vi "event.create_programmatic.request.vi"(4 "Additional Information":T1, 5 "Duration (0s)":dbl, 6 "Properties and Labels":T2, 7 "Time Stamp (now: system time)":timestamp format="%<%x %.3X>T", 8 "error in":errorcluster, 9 "Name":string, 10 "Asset RIDs":string[](array[string])) -> (0 "error out":errorcluster, 3 "request":string)   [LabVIEW 2020, in "Nominal Client.lvclass"]
uses:
  Nominal Client.lvclass
  762c8870-e4d3-421c-a376-3e8bab40d908.vi
  a7848146-fc71-4dc3-8a34-870616c71ff8.vi
  7e86f393-abb9-4d64-98a3-bbc5c32f8c9f.vi
  adfb2873-4f8f-45ec-91b4-e6f8d4ca100d.vi
  f3b2abde-4779-4471-9147-3371a6e54b37.vi
  a6a03f40-2490-4db4-85a0-99c3ddd96217.vi
  <vilib>/LabVIEW Open Source Project/Epoch Date & Time/epoch.UNIX/Epoch.UNIX.lvclass
  C:/Program Files/National Instruments/LabVIEW 2020/vi.lib/LabVIEW Open Source Project/Epoch Date & Time/epoch/Epoch.lvclass
  <vilib>/LabVIEW Open Source Project/Epoch Date & Time/Get Epoch Time.vi
  <vilib>/JDP Science/JSONtext/Variant to JSON Text.vi
  <vilib>/JDP Science/JSONtext/support/Format JSON Object.vi
  <vilib>/JDP Science/JSONtext/LVClass Serializer/JSONtext LVClass Serializer.lvclass
  nominal types/labels/labels.lvclass
  Nominal Client.lvclass/Nominal Client.ctl
  nominal types/properties/properties.lvclass
  <vilib>/JDP Science/JSONtext/JSONtext.lvlib
  133ea0b1-5c8c-48d2-80aa-f88861def257.vi
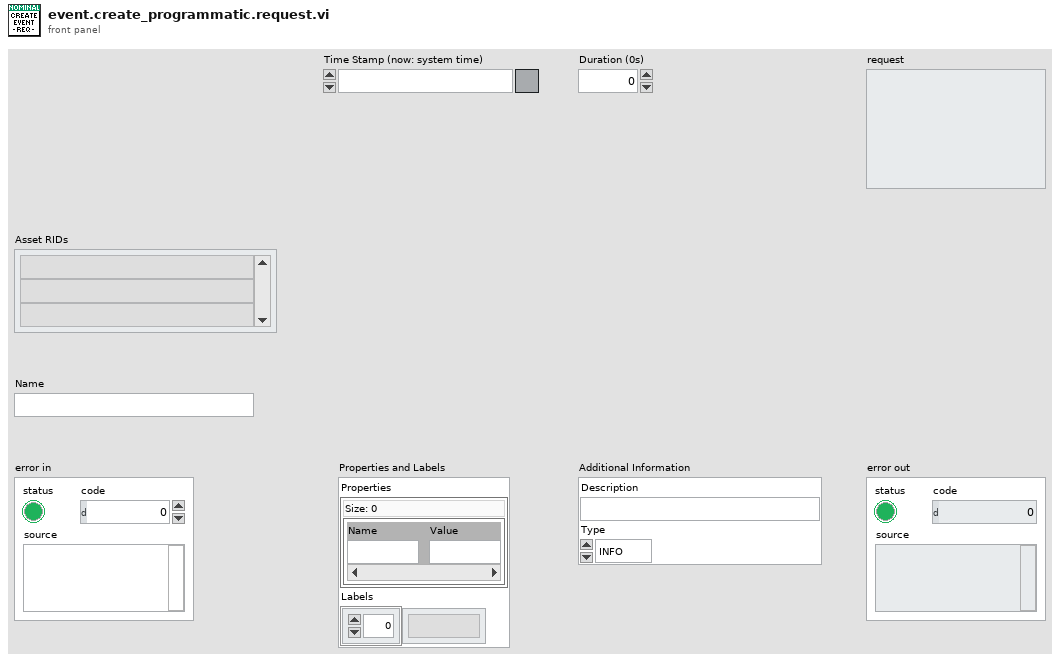
[diagram p1: front panel]
types:
  T1 = cluster{"Description":string, "Type":enum16{"INFO", "FLAG", "ERROR", "SUCCESS"}}
  T2 = cluster{"Properties":map{string, string}, "Labels":string[]}
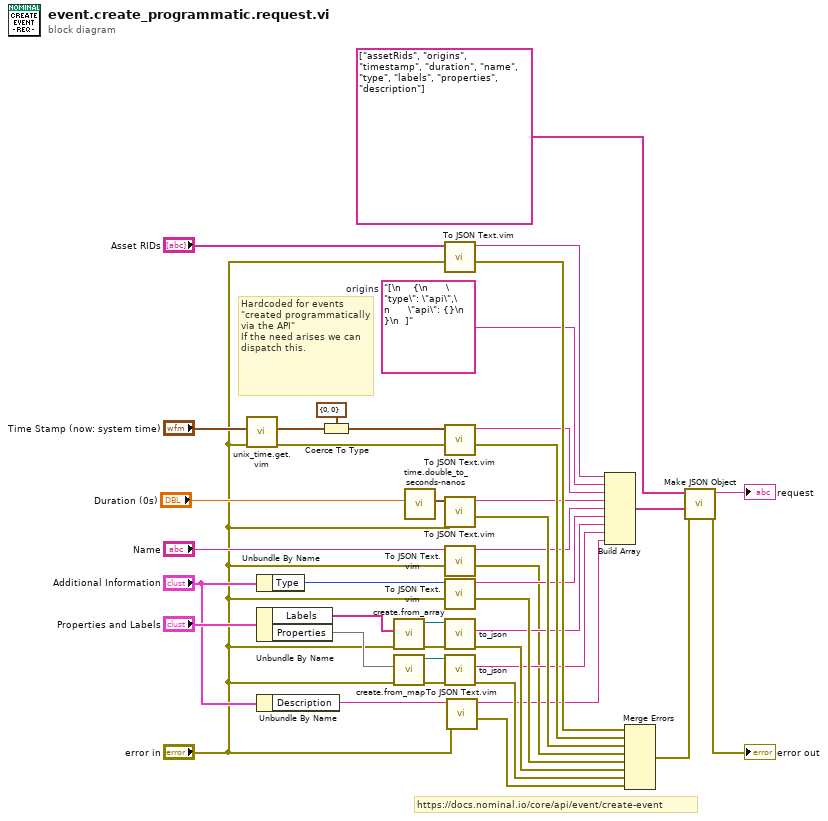
[diagram p0: block diagram]
diagram:
  w22 = "[\n    {\n      \"type\": \"api\",\n      \"api\": {}\n    }\n  ]"  # origins
  # "Hardcoded for events \"created programmatically via the API\"\nIf the need arises we can dispatch this."
  # "https://docs.nominal.io/core/api/event/create-event"
  n1 = call "unix_time.get.vim"("Time Stamp (empty: now) [single or array]"="Time Stamp (now: system time)") -> ("UNIX Timestamp"=w40:cluster{"Seconds":i64, "Nanoseconds":i64})  [unwired: 10 in]
  n2 = Unbundle By Name("Additional Information") -> ("Type"=w6:enum16{"INFO", "FLAG", "ERROR", "SUCCESS"})
  n3 = Unbundle By Name("Properties and Labels") -> ("Labels"=w34:string[], "Properties"=w36:map{string, string})
  n4 = Unbundle By Name("Additional Information") -> ("Description"=w4:string)
  n5 = Coerce To Type(0:w40, 1:cluster{"seconds":i32, "nanos":i32} {"seconds"=0, "nanos"=0} ("UNIX Timestamp")) -> (2:w29:cluster{"seconds":i32, "nanos":i32})
  n6 = call "create.from_array.vi"("error in"="error in", "labels"=w34) -> ("error out"=w32:errorcluster, "labels out"=w33:refnum<class "labels.lvclass">)  [unwired: 8 in]
  n7 = call "create.from_map.vi"("error in"="error in", "properties"=w36) -> ("error out"=w31:errorcluster, "properties out"=w35:refnum<class "properties.lvclass">)  [unwired: 8 in]
  n8 = call "time.double_to_seconds-nanos.vi"("Time (s)"="Duration (0s)") -> ("Seconds Nanos"=w15:cluster{"seconds":i32, "nanos":i32})  [unwired: 10 in]
  n9 = call "To JSON Text.vim"("error in (no error)"="error in", "Anything"="Asset RIDs") -> ("error out"=w27:errorcluster, "<JSON>"=w30:string)  [unwired: 8 in]
  n10 = call "To JSON Text.vim"("error in (no error)"="error in", "Anything"=w29) -> ("error out"=w26:errorcluster, "<JSON>"=w21:string)  [unwired: 8 in]
  n11 = call "To JSON Text.vim"("error in (no error)"="error in", "Anything"=w15) -> ("error out"=w41:errorcluster, "<JSON>"=w14:string)  [unwired: 8 in]
  n12 = call "To JSON Text.vim"("error in (no error)"="error in", "Anything"="Name") -> ("error out"=w13:errorcluster, "<JSON>"=w17:string)  [unwired: 8 in]
  n13 = call "To JSON Text.vim"("error in (no error)"="error in", "Anything"=w6) -> ("error out"=w25:errorcluster, "<JSON>"=w20:string)  [unwired: 8 in]
  n14 = call-dynamic "to_json.vi"("error in"=w32, "labels in"=w33) -> ("error out"=w24:errorcluster, "json"=w19:string)  [unwired: 6 in, 2 out]
  n15 = call-dynamic "to_json.vi"("error in"=w31, "properties in"=w35) -> ("error out"=w23:errorcluster, "json"=w18:string)  [unwired: 6 in, 2 out]
  n16 = call "To JSON Text.vim"("error in (no error)"="error in", "Anything"=w4) -> ("error out"=w2:errorcluster, "<JSON>"=w3:string)  [unwired: 8 in]
  n17 = Build Array(w30, w22, w21, w14, w17, w20, w19, w18, w3) -> (w28:string[])
  n18 = Merge Errors(w27, w26, w41, w13, w25, w24, w23, w2) -> (w16:errorcluster)
  n19 = call <vilib>:"Make JSON Object.vi"("error in (no error)"=w16, "JSON Items"=w28, "Item Names"=string[] ["assetRids", "origins", "timestamp", "duration", "name", "type", "labels", "properties", "description"]) -> ("error out"=→"error out":errorcluster, "<JSON>"=→"request":string)  [unwired: 7 in]
